vi "PPMS.Magnet Status Ring to String.vi"(1 "Field Status":T1 items=["MagnetUnknown"=0, "StablePersistent"=1, "WarmingSwitch"=2, "CoolingSwitch"=3, "StableDriven"=4, "Iterating"=5, "Charging"=6, "Discharging"=7, "CurrentError"=8, "MagnetFailure"=15]) -> (0 "Status String":string)   [LabVIEW 2019, in "instrument.PPMS.lvclass"]
uses:
  instrument.PPMS.lvclass
  Typedefs/PPMS.Magnet Status--ring.ctl
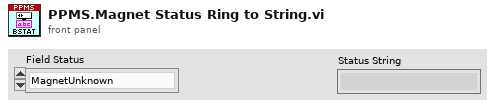
[diagram p1: front panel]
types:
  T1 = typedef "instrument.PPMS.lvclass/PPMS.Magnet Status--ring.ctl" = i32
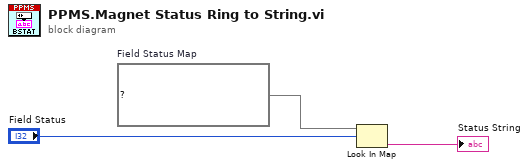
[diagram p0: block diagram]
diagram:
  w1 = map{i32, string} {0="MagnetUnknown", 1="StablePersistent", 2="WarmingSwitch", 3="CoolingSwitch", 4="StableDriven", 5="Iterating", 6="Charging", 7="Discharging", 8="CurrentError", 15="MagnetFailure"}  # Field Status Map
  n1 = Look In Map(map=w1, key="Field Status") -> (value=→"Status String":string)  [unwired: 1 in, 1 out]
